vi "odczytajPrzyspieszenie.vi"(8 "Error In":errorcluster, 10 "Wybór komory":T1, 11 "LINX Resource":T2={"IO"=enum."Remote", "Interface"=enum."TCP", "LINX Device Config"={"Interface"=enum."TCP", "COM Port"="N/A", "TCP Configuration"={"IP Address"="panicattack", "Port"=6999}, "Device Family"=4, "Device ID"=1, "Device Name"="Raspberry Pi Model B", "TCP Ref"=refnum, "Channels"={"DI"=[2, 3, 4, 7, 8, 9, 10, 11, 14, 15, 17, 18, 22, 23, 24, 25, 27], "DO"=[2, 3, 4, 7, 8, 9, 10, 11, 14, 15, 17, 18, 22, 23, 24, 25, 27], "AI"=[], "AO"=[], "PWM"=[], "QE"=[], "UART"=[0], "I2C 2"=[0, 1], "SPI"=[0], "CAN"=[], "Servo"=[], "AI Ref (V)"=0.0, "AI Resolution (Bits)"=0, "AO Ref (V)"=0.0, "AO Resolution (Bits)"=0}}}) -> (0 "Error Out":errorcluster, 2 "K¹ty nachylenia (st.)":dbl[](array[numeric]), 3 "LINX Resource 2":T2)   [LabVIEW 2014]
uses:
  <vilib>/MakerHub/LINX/Private/Type Defs/LINX Ref.ctl
  <vilib>/MakerHub/LINX/Private/Type Defs/Platform.ctl
  <vilib>/MakerHub/LINX/Private/Type Defs/Interface.ctl
  <vilib>/MakerHub/LINX/Private/Device/Type Defs/LINX Device Config.ctl
  <vilib>/MakerHub/LINX/Private/Device/Type Defs/TCP Config.ctl
  <vilib>/MakerHub/LINX/Private/Device/Type Defs/Channels.ctl
  parametryKomorVIs/WyborKomory.ctl
  <vilib>/MakerHub/LINX/LMH-LINX.lvlib
  <vilib>/MakerHub/LINX/Private/Device/Device.lvlib
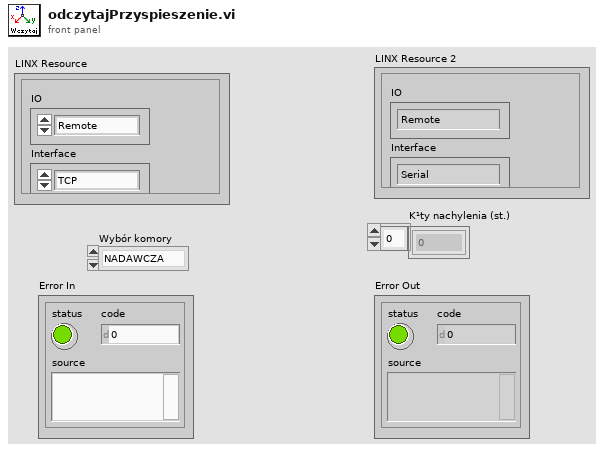
[diagram p1: front panel]
types:
  T1 = typedef "WyborKomory.ctl" = enum16{"NADAWCZA", "ODBIORCZA"}
  T2 = typedef "LMH-LINX.lvlib/LINX Ref.ctl" = cluster{"IO":T3, "Interface":T4, "LINX Device Config":T5}
  T3 = typedef "LMH-LINX.lvlib/Platform.ctl" = enum16{"Remote", "Local"}
  T4 = typedef "LMH-LINX.lvlib/Interface.ctl" = enum16{"Serial", "TCP"}
  T5 = typedef "LMH-LINX.lvlib/Device.lvlib/LINX Device Config.ctl" = cluster{"Interface":T4, "COM Port":refnum<visa-resource-name>, "TCP Configuration":T6, "Device Family":u8, "Device ID":u8, "Device Name":string, "TCP Ref":refnum<k5>, "Channels":T7}
  T6 = typedef "LMH-LINX.lvlib/Device.lvlib/TCP Config.ctl" = cluster{"IP Address":string, "Port":u16}
  T7 = typedef "LMH-LINX.lvlib/Channels.ctl" = cluster{"DI":u8[], "DO":u8[], "AI":u8[], "AO":u8[], "PWM":u8[], "QE":u8[], "UART":u8[], "I2C 2":u8[], "SPI":u8[], "CAN":u8[], "Servo":u8[], "AI Ref (V)":dbl, "AI Resolution (Bits)":u8, "AO Ref (V)":dbl, "AO Resolution (Bits)":u8}
  T8 = typedef "PinoutLista.ctl" = cluster{"LEWO":u8, "PRAWO":u8, "GÓRA":u8, "Dӣ":u8, "CZUJNIK":u8, "I2C ADRES":u8}
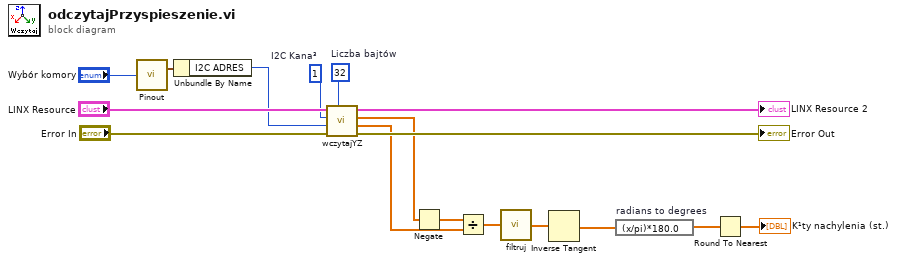
[diagram p0: block diagram]
diagram:
  w4 = u8 1  # I2C Kana³
  w6 = u8 32  # Liczba bajtów
  n1 = call "Pinout.vi"("Wybór komory"="Wybór komory") -> ("Wyjœcie"=w3:T8)  [unwired: 4 in]
  n2 = Unbundle By Name(w3) -> ("I2C ADRES"=w1:u8)
  n3 = call "wczytajYZ.vi"("Liczba bajtów"=w6, "error in (no error)"="Error In", "I2C Adres"=w1, "I2C Kana³"=w4, "LINX Resource in"="LINX Resource") -> ("error out"=→"Error Out":errorcluster, "Oœ Z"=w10:dbl[], "Oœ Y"=w11:dbl[], "LINX Resource out"=→"LINX Resource 2":T2)  [unwired: 3 in]
  n4 = Negate(x=w11) -> (-x=w12:dbl[])
  n5 = Divide(x=w12, y=w10) -> (x/y=w8:dbl[])
  n6 = call "filtruj.vi"("tab. wejœciowa"=w8) -> ("tab. przefiltrowana"=w7:dbl[])  [unwired: 4 in]
  n7 = Inverse Tangent(1:w7) -> (0:w13:dbl[])
  n8 = expression code="(x/pi)*180.0" "radians to degrees"(w13) -> (w14:dbl[])
  n9 = Round To Nearest(number=w14) -> (nearest integer value=→"K¹ty nachylenia (st.)":dbl[])
